vi "Configure Measurement (Resistance).vi"(0 "VISA resource name":refnum<visa-resource-name>, 1 "Channel (0: Channel 1)":i32(ring) items=["Channel 1", "Channel 2"], 3 "Resistance Range (2 Ohm)":dbl=2.0, 4 "Resistance Measurement Mode (1: Auto)":i32(ring)=1 items=["Manual", "Auto"], 5 "error in (no error)":errorcluster, 6 "Auto Resistance NPLC (F: Disable)":bool, 7 "Resistance NPLC (0.1)":dbl=0.1, 8 "Enable Resistance Compensation (F: Disable)":bool, 9 "Resistance Range Upper Limit (2E+8 Ohm)":dbl=200000000.0, 10 "Resistance Auto Range (T: Enable)":bool=TRUE, 11 "Resistance Range Lower Limit (2 Ohm)":dbl=2.0) -> (14 "VISA resource name out":refnum<visa-resource-name>, 19 "error out":errorcluster)   [LabVIEW 2020, in "Agilent B2900 Series.lvlib"]
doc: "Change settings for resistance measurement function.\n\n<B>Note:</B>\nCommands in default part of the case structure are not applicable for Agilent models B2961A, B2962A, B2961B,B2962B,B2961C and B2962C."
uses:
  Agilent B2900 Series.lvlib
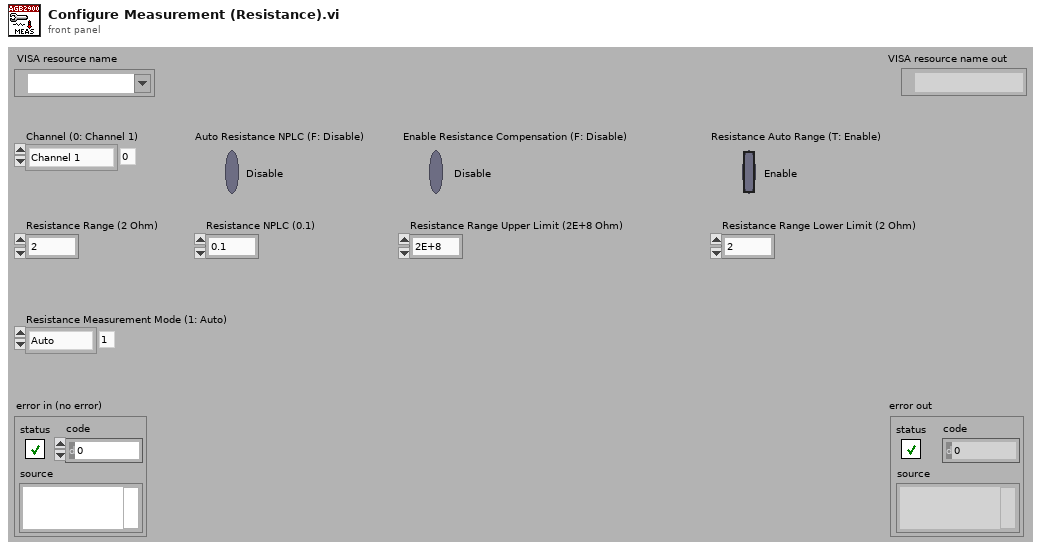
[diagram p1: front panel]
types:
  T1 = typedef "Agilent B2900 Series.lvlib/Extended User Data.ctl" = cluster{"B2900 Series Mode":u16}
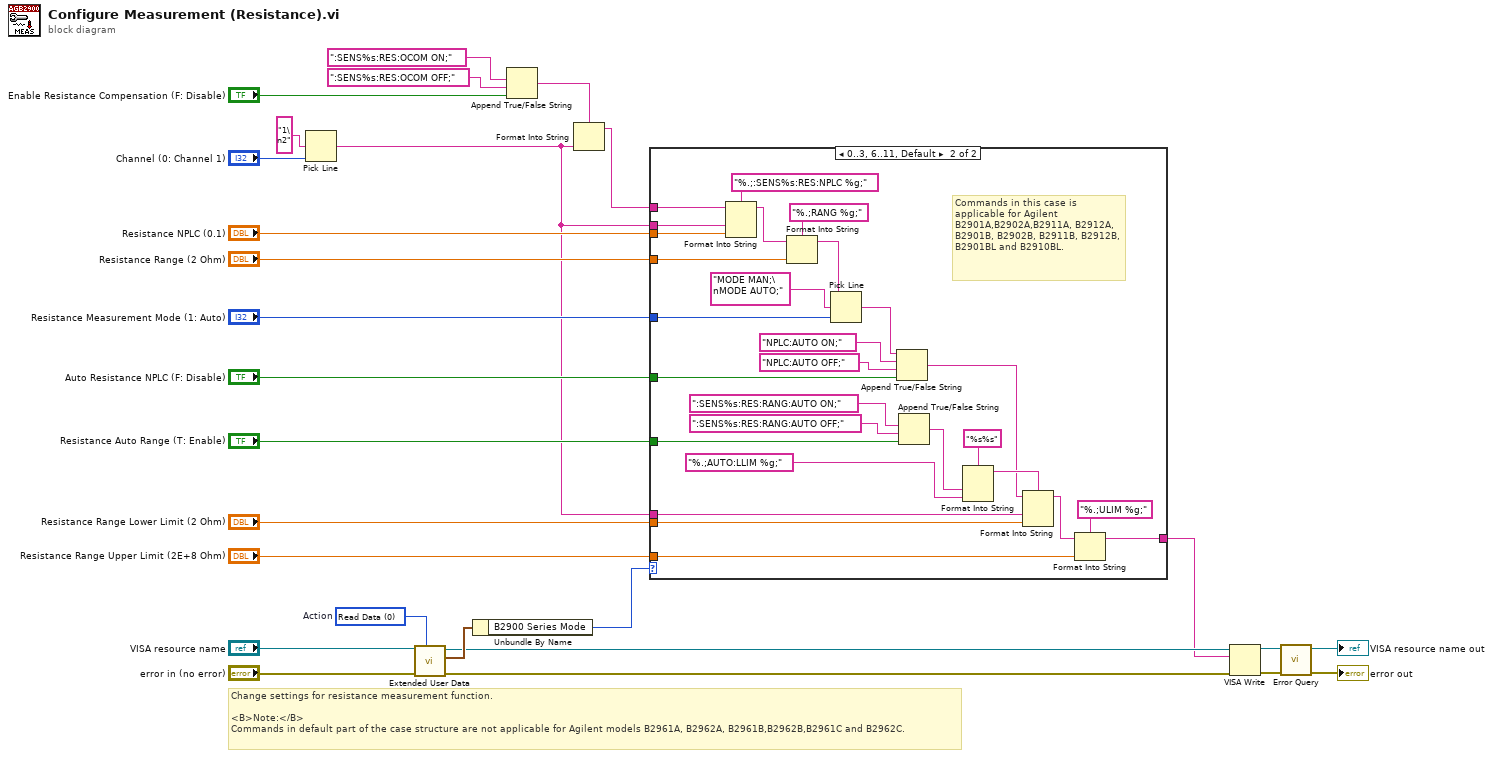
[diagram p0: block diagram]
diagram:
  w18 = 0 items=["Read Data", "Write Data", "Clear Data", "Clear ALL Data"]  # Action
  # "Change settings for resistance measurement function.\n\n<B>Note:</B>\nCommands in default part of the case structure are not applicable for Agilent models B2961A, B2962A, B2961B,B2962B,B2961C and B2962C."
  n1 = Pick Line(multi-line string="1\n2" ("string (\"\")"), line index="Channel (0: Channel 1)") -> (output string=w6:string)  [unwired: 1 in]
  n2 = call "Extended User Data.vi"("Action (1: Write Data)"=w18, "Error In (no error)"="error in (no error)", "VISA resource name in"="VISA resource name") -> ("Error Out"=w13:errorcluster, "User Data Out"=w17:T1, "VISA resource name out"=w14:refnum<visa-resource-name>)  [unwired: 6 in]
  n3 = Unbundle By Name(w17) -> ("B2900 Series Mode"=w12:u16)
  n4 = Append True/False String(1:"Enable Resistance Compensation (F: Disable)", 2:":SENS%s:RES:OCOM OFF;", 3:":SENS%s:RES:OCOM ON;") -> (0:w1:string)  [unwired: 1 in]
  n5 = Format Into String(format string=w1, w6) -> (resulting string=w2:string)  [unwired: 2 in, 1 out]
  n6 = case shown="0..3, 6..11, Default" w12 {
    tunnel: w6 -> [_ w39]
    tunnel: "Resistance Range (2 Ohm)" -> [_ w38]
    tunnel: "Resistance NPLC (0.1)" -> [_ w37]
    tunnel: "Resistance Measurement Mode (1: Auto)" -> [_ w36]
    tunnel: "Auto Resistance NPLC (F: Disable)" -> [_ w35]
    tunnel: "Resistance Auto Range (T: Enable)" -> [_ w34]
    tunnel: w6 -> [_ w33]
    tunnel: "Resistance Range Lower Limit (2 Ohm)" -> [_ w32]
    tunnel: "Resistance Range Upper Limit (2E+8 Ohm)" -> [_ w31]
    tunnel: [w28 w30] -> w3
    tunnel: w2 -> [w28 w29]
    frame 4, 5, 12, 13 {
      # "Commands in this case are\napplicable for Agilent B2961A,B2962A, B2961B, B2962B."
    }
    frame 0..3, 6..11, Default {
      # "Commands in this case is applicable for Agilent B2901A,B2902A,B2911A, B2912A, B2901B, B2902B, B2911B, B2912B, B2901BL and B2910BL."
      n7 = Format Into String(format string="%.;:SENS%s:RES:NPLC %g;", initial string=w29, w39, w37) -> (resulting string=w43:string)  [unwired: 1 in, 1 out]
      n8 = Format Into String(format string="%.;RANG %g;", initial string=w43, w38) -> (resulting string=w46:string)  [unwired: 1 in, 1 out]
      n9 = Pick Line(string ("")=w46, multi-line string="MODE MAN;\nMODE AUTO;", line index=w36) -> (output string=w56:string)
      n10 = Append True/False String(1:w35, 2:"NPLC:AUTO OFF;", 3:"NPLC:AUTO ON;", 4:w56) -> (0:w50:string)
      n11 = Append True/False String(1:w34, 2:":SENS%s:RES:RANG:AUTO OFF;", 3:":SENS%s:RES:RANG:AUTO ON;") -> (0:w52:string)  [unwired: 1 in]
      n12 = Format Into String(format string="%s%s", w52, "%.;AUTO:LLIM %g;") -> (resulting string=w54:string)  [unwired: 2 in, 1 out]
      n13 = Format Into String(format string=w54, initial string=w50, w33, w32) -> (resulting string=w49:string)  [unwired: 1 in, 1 out]
      n14 = Format Into String(format string="%.;ULIM %g;", initial string=w49, w31) -> (resulting string=w30:string)  [unwired: 1 in, 1 out]
    }
  }
  n15 = VISA Write(VISA resource name=w14, write buffer=w3, error in (no error)=w13) -> (VISA resource name out=w24:refnum<visa-resource-name>, error out=w23:errorcluster)  [unwired: 1 out]
  n16 = call "Error Query.vi"("error in (no error)"=w23, "VISA resource name"=w24) -> ("error out"=→"error out":errorcluster, "VISA resource name out"=→"VISA resource name out":refnum<visa-resource-name>)  [unwired: 6 in, 2 out]
